vi "cut_off_gravity_factor_from_acc.vi"() -> ()   [LabVIEW 2015]
panel:
  out "A_z":dbl
  out "A_y":dbl
  out "A_x":dbl
  in  "stop":bool
  in  "Az":i32(slide) scale=-2000.0..2000.0
  in  "Ay":i32(slide) scale=-2000.0..2000.0
  in  "Ax":i32(slide) scale=-2000.0..2000.0
  # "1000 = 1g"
  # "Vi is cutting off the constant component from the \nMPU-6050's accelrameter readings"
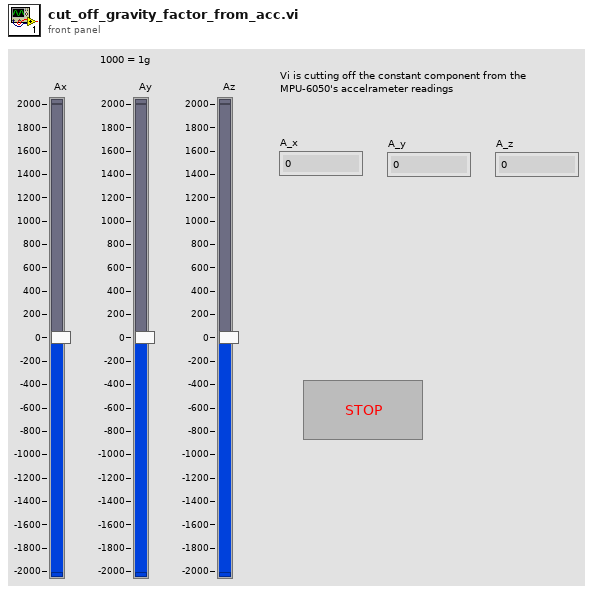
[diagram p1: front panel]
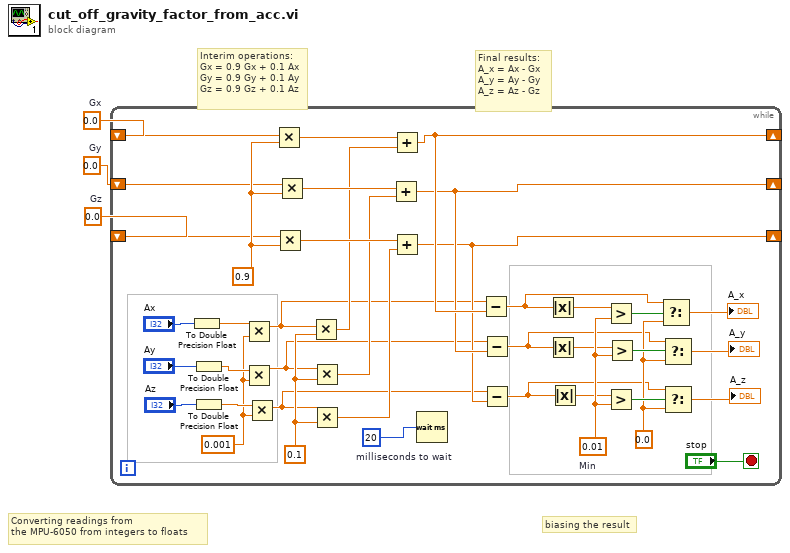
[diagram p0: block diagram]
diagram:
  w1 = 0.0  # Gz
  w2 = 0.0  # Gy
  w3 = 0.0  # Gx
  # "biasing the result"
  # "Final results:\nA_x = Ax - Gx\nA_y = Ay - Gy\nA_z = Az - Gz"
  # "Interim operations:\nGx = 0.9 Gx + 0.1 Ax\nGy = 0.9 Gy + 0.1 Ay\nGz = 0.9 Gz + 0.1 Az"
  # "Converting readings from \nthe MPU-6050 from integers to floats"
  n1 = while {
    shift-right: [w28] -> _
    shift-left: w3 -> [w31]
    shift-right: [w27] -> _
    shift-left: w2 -> [w30]
    shift-right: [w26] -> _
    shift-left: w1 -> [w29]
    stop <- "stop" stop-if-true
    w10 = 0.0 ("t")
    w17 = 0.01  # Min
    w18 = 0.001 ("y")
    w40 = 0.1 ("y")
    w41 = 0.9 ("y")
    w42 = u32 20  # milliseconds to wait
    n2 = To Double Precision Float(number="Ax") -> (double precision float=w21:dbl)
    n3 = To Double Precision Float(number="Ay") -> (double precision float=w20:dbl)
    n4 = To Double Precision Float(number="Az") -> (double precision float=w19:dbl)
    n5 = Multiply(x=w21, y=w18) -> (x*y=w25:dbl)
    n6 = Multiply(x=w20, y=w18) -> (x*y=w24:dbl)
    n7 = Multiply(x=w19, y=w18) -> (x*y=w23:dbl)
    n8 = Multiply(x=w31, y=w41) -> (x*y=w39:dbl)
    n9 = Multiply(x=w29, y=w41) -> (x*y=w37:dbl)
    n10 = Multiply(x=w30, y=w41) -> (x*y=w38:dbl)
    n11 = Multiply(x=w25, y=w40) -> (x*y=w36:dbl)
    n12 = Multiply(x=w24, y=w40) -> (x*y=w35:dbl)
    n13 = Multiply(x=w23, y=w40) -> (x*y=w34:dbl)
    n14 = Add(x=w38, y=w35) -> (x+y=w27:dbl)
    n15 = Add(x=w39, y=w36) -> (x+y=w28:dbl)
    n16 = Add(x=w37, y=w34) -> (x+y=w26:dbl)
    n17 = Wait (ms)(milliseconds to wait=w42) -> ()  [unwired: 1 out]
    n18 = Subtract(x=w25, y=w28) -> (x-y=w9:dbl)
    n19 = Subtract(x=w24, y=w27) -> (x-y=w8:dbl)
    n20 = Subtract(x=w23, y=w26) -> (x-y=w7:dbl)
    n21 = Absolute Value(x=w9) -> (abs(x)=w5:dbl)
    n22 = Absolute Value(x=w8) -> (abs(x)=w6:dbl)
    n23 = Absolute Value(x=w7) -> (abs(x)=w4:dbl)
    n24 = Greater?(x=w5, y=w17) -> (0:w16:bool)
    n25 = Greater?(x=w4, y=w17) -> (0:w14:bool)
    n26 = Greater?(x=w6, y=w17) -> (0:w15:bool)
    n27 = Select(t=w9, s=w16, f=w10) -> (s? t:f=→"A_x":dbl)
    n28 = Select(t=w8, s=w15, f=w10) -> (s? t:f=→"A_y":dbl)
    n29 = Select(t=w7, s=w14, f=w10) -> (s? t:f=→"A_z":dbl)
  }
